vi "KG set spump syringe.vi"(8 "Fehler (Eingang, kein Fehler)":errorcluster, 9 "density":dbl, 10 "pump":u32, 11 "VISA-Ressourcenname":refnum<visa-resource-name>) -> (0 "Fehler (Ausgang)":errorcluster, 2 "Kommando gesendet":string, 3 "VISA-Ressourcenname (Ausgang)":refnum<visa-resource-name>)   [LabVIEW 2020, in "Linearisierung v2.lvlib" / "Gasteiler.lvlib" / "HovaCAL_Interface.lvlib" / "KGN.lvlib" / "set.lvlib"]
uses:
  set.lvlib
  KGN.lvlib
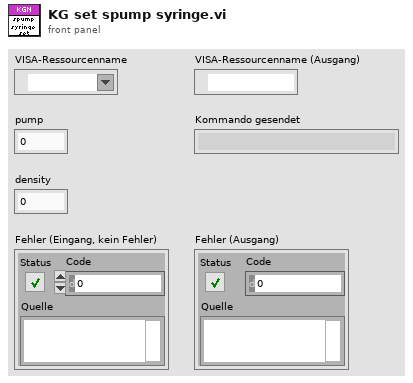
[diagram p1: front panel]
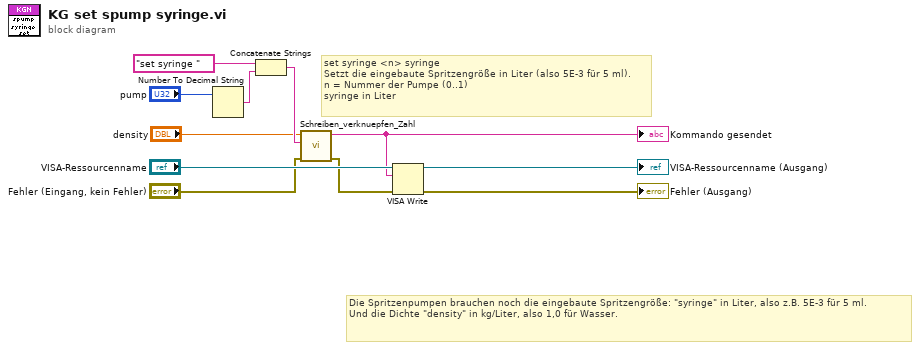
[diagram p0: block diagram]
diagram:
  # "Die Spritzenpumpen brauchen noch die eingebaute Spritzengröße: \"syringe\" in Liter, also z.B. 5E-3 für 5 ml.\nUnd die Dichte \"density\" in kg/Liter, also 1,0 für Wasser."
  # "set syringe <n> syringe\nSetzt die eingebaute Spritzengröße in Liter (also 5E-3 für 5 ml).\nn = Nummer der Pumpe (0..1)\nsyringe in Liter"
  n1 = Number To Decimal String(number="pump") -> (decimal integer string=w2:string)  [unwired: 1 in]
  n2 = Concatenate Strings("set syringe " ("Schreibpuffer"), w2) -> (w3:string)
  n3 = call "Schreiben_verknuepfen_Zahl.vi"("error in (no error)"="Fehler (Eingang, kein Fehler)", "Order"=w3, "Zahl"="density") -> ("error out"=w6:errorcluster, "Verknüpfter String"=w5:string)  [unwired: 7 in]
  "Kommando gesendet" <- w5
  n4 = VISA Write(VISA resource name="VISA-Ressourcenname", write buffer=w5, error in (no error)=w6) -> (VISA resource name out=→"VISA-Ressourcenname (Ausgang)":refnum<visa-resource-name>, error out=→"Fehler (Ausgang)":errorcluster)  [unwired: 1 out]
